vi "Get EDS.vi"(10 "Path":path, 11 "UI Actor in":refnum<class "UI Actor.lvclass">) -> (2 "EDS":refnum<class "Electronic Datasheet.lvclass">, 3 "UI Actor out":refnum<class "UI Actor.lvclass">)   [LabVIEW 2019, in "UI Actor.lvlib" / "UI Actor.lvclass"]
uses:
  UI Actor.lvclass
  UI Actor.lvclass/UI Actor.ctl
  Electronic Datasheet/Electronic Datasheet.lvclass
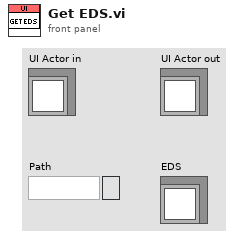
[diagram p1: front panel]
types:
  T1 = map{path, refnum<class "Electronic Datasheet.lvclass">}
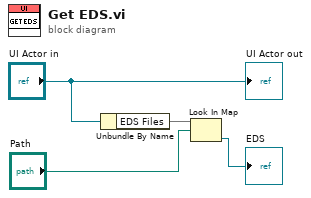
[diagram p0: block diagram]
diagram:
  n1 = Unbundle By Name("UI Actor in") -> ("EDS Files"=w3:T1)
  n2 = Look In Map(map=w3, key="Path") -> (value=→"EDS":refnum<class "Electronic Datasheet.lvclass">)  [unwired: 1 in, 1 out]
  "UI Actor out" <- "UI Actor in"
